vi "Nfocus driver V0.3.vi"(5 "error in":errorcluster) -> (0 "error out":errorcluster)   [LabVIEW 2016]
panel:
  in  "Refs In":T1
  out "Running":bool
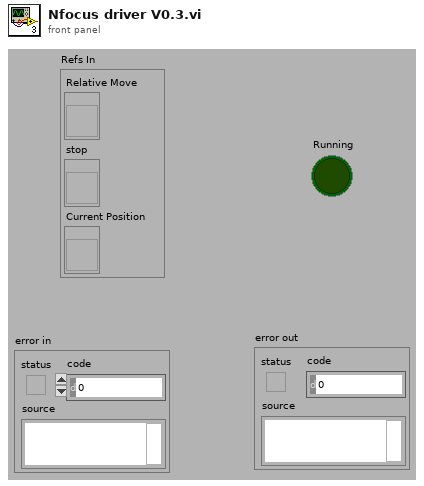
[diagram p1: front panel]
types:
  T1 = cluster{"Relative Move":refnum<vi>, "stop":refnum<vi>, "Current Position":refnum<vi>}
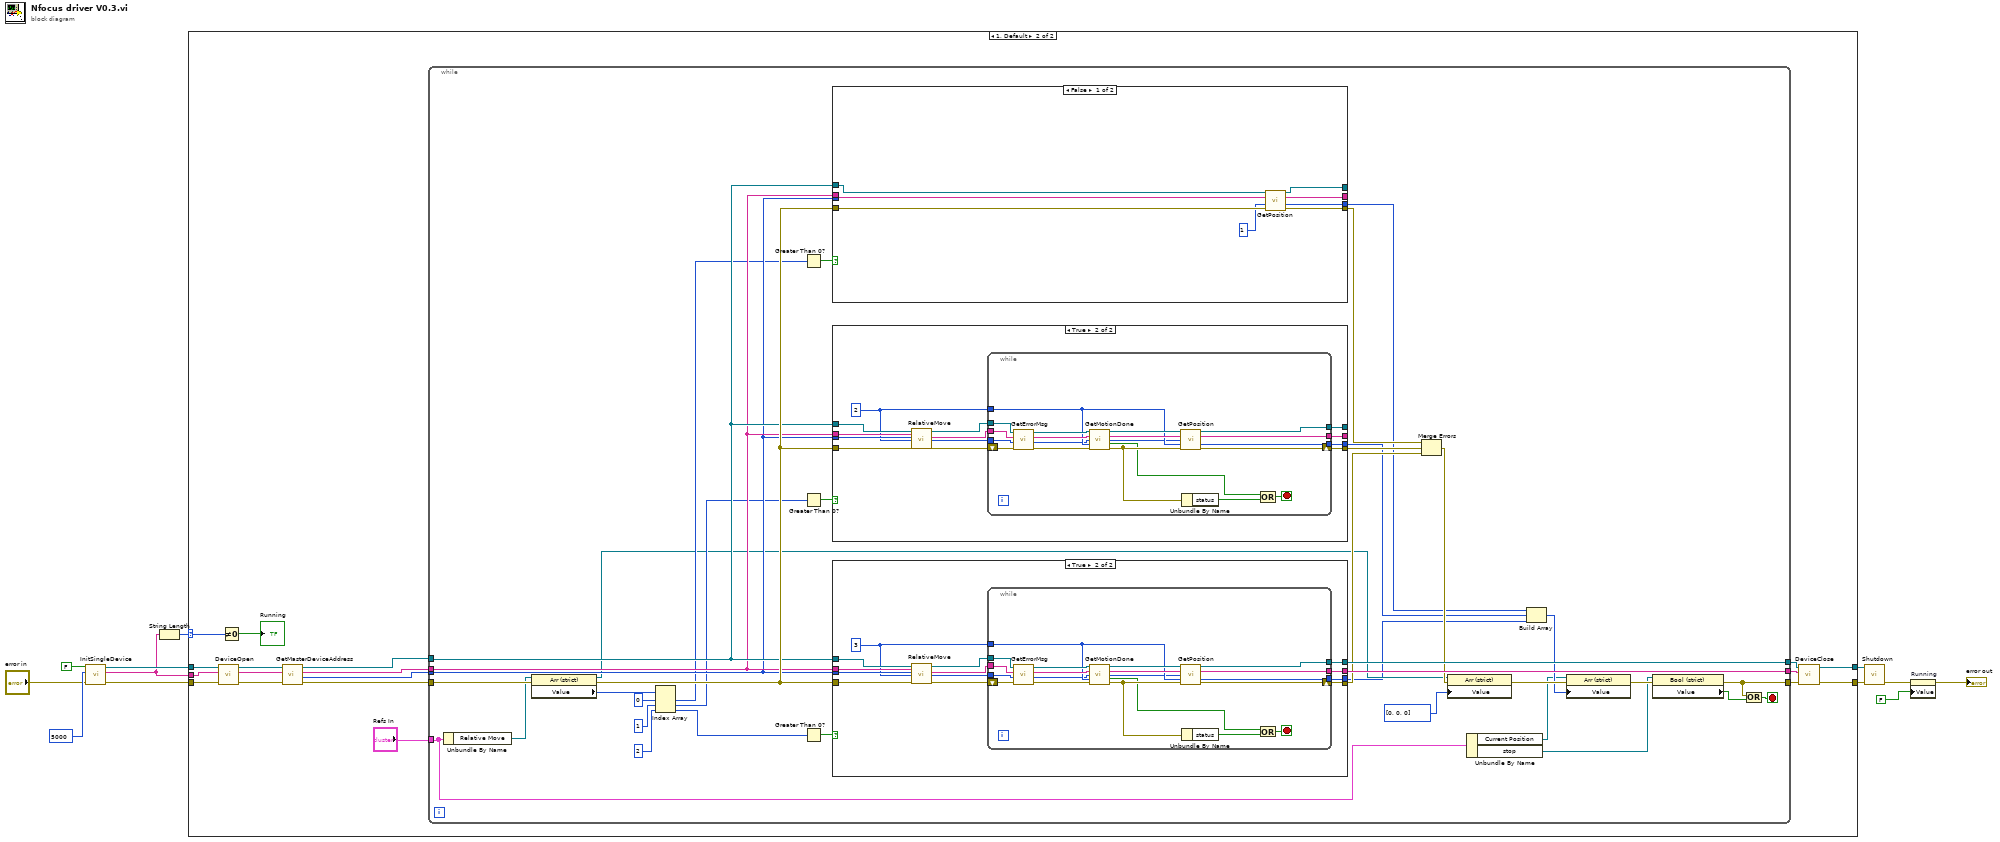
[diagram p0: block diagram]
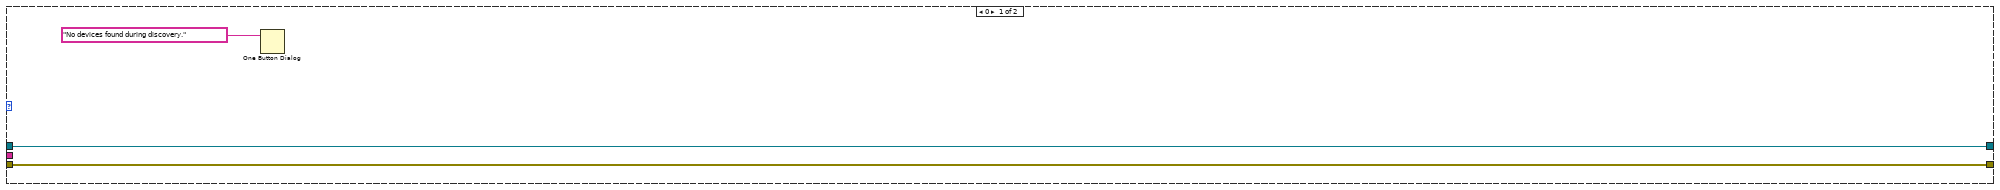
[diagram p2: hidden frame]
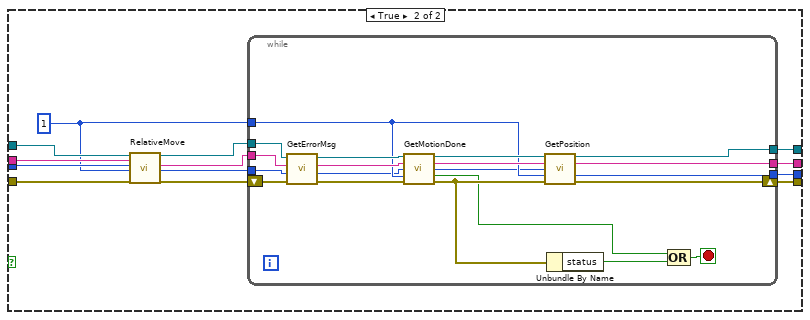
[diagram p3: hidden frame]
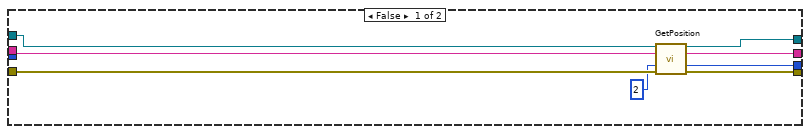
[diagram p4: hidden frame]
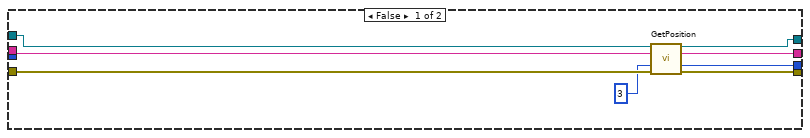
[diagram p5: hidden frame]
diagram:
  n1 = call "InitSingleDevice.vi"("error in (no error)"="error in", "msecDelayForDiscovery"=5000, "logging"=FALSE) -> ("error out"=w5:errorcluster, "DeviceKey Out"=w6:string, "CmdLib Out"=w8:refnum<k24>)  [unwired: 2 in]
  n2 = String Length(string=w6) -> (length=w7:i32)
  n3 = case shown="1, Default" w7 {
    selector: w7 -> [_ w18]
    tunnel: [w14 w20] -> w10
    tunnel: [w13 w22] -> w9
    tunnel: w8 -> [w14 w26]
    tunnel: w6 -> [_ w28]
    tunnel: w5 -> [w13 w30]
    frame 0 {
      n4 = One Button Dialog(message="No devices found during discovery.") -> ()  [unwired: 1 in, 1 out]
    }
    frame 1, Default {
      n5 = call "DeviceOpen.vi"("error in (no error)"=w30, "DeviceKey In"=w28, "CmdLib In"=w26) -> ("error out"=w29:errorcluster, "DeviceKey Out"=w27:string, "CmdLib Out"=w25:refnum<k24>)  [unwired: 2 in]
      n6 = Not Equal To 0?(x=w18) -> (x != 0?=→"Running":bool)
      n7 = call "GetMasterDeviceAddress.vi"("error in (no error)"=w29, "DeviceKey In"=w27, "CmdLib In"=w25) -> ("error out"=w19:errorcluster, "Device Address"=w33:i32, "DeviceKey Out"=w31:string, "CmdLib Out"=w32:refnum<k24>)  [unwired: 1 in]
      n8 = while {
        tunnel: w33 -> [w57]
        tunnel: w32 -> [w59]
        tunnel: [w68] -> w21
        tunnel: w19 -> [w61]
        tunnel: [w66] -> w23
        tunnel: w31 -> [w58]
        tunnel: [w69] -> w24
        tunnel: "Refs In" -> [w36]
        stop <- w67 stop-if-true
        n9 = Unbundle By Name(w36) -> ("Relative Move"=w46:refnum<vi>)
        n10 = property class="Arr (strict)"(reference=w46, error in=w61) -> (reference out=w44:refnum<vi>, error out=w60:errorcluster, "Value"=w63:i32[])
        n11 = Index Array(array=w63, index #1=0 ("index"), index #2=1 ("index"), index #3=2 ("index")) -> (element #1=w52:i32, element #2=w51:i32, element #3=w50:i32)
        n12 = Greater Than 0?(x=w52) -> (x > 0?=w53:bool)
        n13 = Greater Than 0?(x=w51) -> (x > 0?=w54:bool)
        n14 = Greater Than 0?(x=w50) -> (x > 0?=w64:bool)
        n15 = case shown="False" w53 {
          tunnel: w57 -> [_ w90]
          tunnel: w59 -> [w77 w89]
          tunnel: w58 -> [w76 w88]
          tunnel: [w73 w87] -> _
          tunnel: [w72 w86] -> _
          tunnel: w60 -> [w75 w85]
          tunnel: [w74 w84] -> w49
          tunnel: [w71 w78] -> w40
          frame False {
            n16 = call "GetPosition.vi"("CmdLib In"=w77, "DeviceKey In"=w76, "Motor"=1, "error in (no error)"=w75) -> ("CmdLib Out"=w72:refnum<k24>, "DeviceKey Out"=w73:string, "Position"=w71:i32, "error out"=w74:errorcluster)  [unwired: 7 in, 1 out]
          }
          frame True {
            w79 = 1
            n17 = call "RelativeMove.vi"("CmdLib In"=w89, "DeviceKey In"=w88, "Device Address In"=w90, "Motor"=w79, "error in (no error)"=w85) -> ("CmdLib Out"=w83:refnum<k24>, "DeviceKey Out"=w82:string, "Device Address Out"=w80:i32, "error out"=w81:errorcluster)  [unwired: 11 in]
            n18 = while {
              tunnel: w79 -> [w106]
              tunnel: w83 -> [w105]
              tunnel: w82 -> [w104]
              tunnel: [w99] -> w86
              tunnel: w80 -> [w98]
              shift-right: [w100] -> w84
              shift-left: w81 -> [w103]
              tunnel: [w95] -> w87
              tunnel: [w91] -> w78
              stop <- w94 stop-if-true
              n19 = call "GetErrorMsg.vi"("error in (no error)"=w103, "Device Address In"=w98, "DeviceKey In"=w104, "CmdLib In"=w105) -> ("error out"=w102:errorcluster, "Device Address Out"=w97:i32, "DeviceKey Out"=w108:string, "CmdLib Out"=w107:refnum<k24>)
              n20 = call "GetMotionDone.vi"("CmdLib In"=w107, "DeviceKey In"=w108, "Device Address In"=w97, "Motor"=w106, "error in (no error)"=w102) -> ("CmdLib Out"=w109:refnum<k24>, "DeviceKey Out"=w110:string, "Device Address Out"=w96:i32, "Is Motion Done"=w93:bool, "error out"=w101:errorcluster)  [unwired: 6 in]
              n21 = call "GetPosition.vi"("CmdLib In"=w109, "DeviceKey In"=w110, "Device Address In"=w96, "Motor"=w106, "error in (no error)"=w101) -> ("CmdLib Out"=w99:refnum<k24>, "DeviceKey Out"=w95:string, "Position"=w91:i32, "error out"=w100:errorcluster)  [unwired: 6 in, 1 out]
              n22 = Unbundle By Name(w101) -> ("status"=w92:bool)
              n23 = Compound Arithmetic op=OR(w93, w92) -> (w94:bool)
            }
          }
        }
        n24 = case shown="True" w54 {
          tunnel: w57 -> [_ w131]
          tunnel: w59 -> [w118 w130]
          tunnel: w58 -> [w117 w129]
          tunnel: [w114 w128] -> _
          tunnel: [w115 w127] -> _
          tunnel: w60 -> [w116 w126]
          tunnel: [w113 w125] -> w48
          tunnel: [w111 w119] -> w39
          frame False {
            n25 = call "GetPosition.vi"("CmdLib In"=w118, "DeviceKey In"=w117, "Motor"=2, "error in (no error)"=w116) -> ("CmdLib Out"=w115:refnum<k24>, "DeviceKey Out"=w114:string, "Position"=w111:i32, "error out"=w113:errorcluster)  [unwired: 7 in, 1 out]
          }
          frame True {
            w120 = 2
            n26 = call "RelativeMove.vi"("CmdLib In"=w130, "DeviceKey In"=w129, "Device Address In"=w131, "Motor"=w120, "error in (no error)"=w126) -> ("CmdLib Out"=w124:refnum<k24>, "DeviceKey Out"=w123:string, "Device Address Out"=w121:i32, "error out"=w122:errorcluster)  [unwired: 11 in]
            n27 = while {
              tunnel: w120 -> [w147]
              tunnel: w124 -> [w146]
              tunnel: w123 -> [w145]
              tunnel: [w140] -> w127
              tunnel: w121 -> [w139]
              shift-right: [w141] -> w125
              shift-left: w122 -> [w144]
              tunnel: [w136] -> w128
              tunnel: [w132] -> w119
              stop <- w135 stop-if-true
              n28 = call "GetErrorMsg.vi"("error in (no error)"=w144, "Device Address In"=w139, "DeviceKey In"=w145, "CmdLib In"=w146) -> ("error out"=w143:errorcluster, "Device Address Out"=w138:i32, "DeviceKey Out"=w149:string, "CmdLib Out"=w148:refnum<k24>)
              n29 = call "GetMotionDone.vi"("CmdLib In"=w148, "DeviceKey In"=w149, "Device Address In"=w138, "Motor"=w147, "error in (no error)"=w143) -> ("CmdLib Out"=w150:refnum<k24>, "DeviceKey Out"=w151:string, "Device Address Out"=w137:i32, "Is Motion Done"=w134:bool, "error out"=w142:errorcluster)  [unwired: 6 in]
              n30 = call "GetPosition.vi"("CmdLib In"=w150, "DeviceKey In"=w151, "Device Address In"=w137, "Motor"=w147, "error in (no error)"=w142) -> ("CmdLib Out"=w140:refnum<k24>, "DeviceKey Out"=w136:string, "Position"=w132:i32, "error out"=w141:errorcluster)  [unwired: 6 in, 1 out]
              n31 = Unbundle By Name(w142) -> ("status"=w133:bool)
              n32 = Compound Arithmetic op=OR(w134, w133) -> (w135:bool)
            }
          }
        }
        n33 = case shown="True" w64 {
          tunnel: w57 -> [_ w172]
          tunnel: w59 -> [w159 w171]
          tunnel: w58 -> [w158 w170]
          tunnel: [w155 w169] -> w69
          tunnel: [w154 w168] -> w68
          tunnel: w60 -> [w157 w167]
          tunnel: [w156 w166] -> w47
          tunnel: [w152 w160] -> w38
          frame False {
            n34 = call "GetPosition.vi"("CmdLib In"=w159, "DeviceKey In"=w158, "Motor"=3, "error in (no error)"=w157) -> ("CmdLib Out"=w154:refnum<k24>, "DeviceKey Out"=w155:string, "Position"=w152:i32, "error out"=w156:errorcluster)  [unwired: 7 in, 1 out]
          }
          frame True {
            w161 = 3
            n35 = call "RelativeMove.vi"("CmdLib In"=w171, "DeviceKey In"=w170, "Device Address In"=w172, "Motor"=w161, "error in (no error)"=w167) -> ("CmdLib Out"=w165:refnum<k24>, "DeviceKey Out"=w164:string, "Device Address Out"=w162:i32, "error out"=w163:errorcluster)  [unwired: 11 in]
            n36 = while {
              tunnel: w161 -> [w188]
              tunnel: w165 -> [w187]
              tunnel: w164 -> [w186]
              tunnel: [w181] -> w168
              tunnel: w162 -> [w180]
              shift-right: [w182] -> w166
              shift-left: w163 -> [w185]
              tunnel: [w177] -> w169
              tunnel: [w173] -> w160
              stop <- w176 stop-if-true
              n37 = call "GetErrorMsg.vi"("error in (no error)"=w185, "Device Address In"=w180, "DeviceKey In"=w186, "CmdLib In"=w187) -> ("error out"=w184:errorcluster, "Device Address Out"=w179:i32, "DeviceKey Out"=w190:string, "CmdLib Out"=w189:refnum<k24>)
              n38 = call "GetMotionDone.vi"("CmdLib In"=w189, "DeviceKey In"=w190, "Device Address In"=w179, "Motor"=w188, "error in (no error)"=w184) -> ("CmdLib Out"=w191:refnum<k24>, "DeviceKey Out"=w192:string, "Device Address Out"=w178:i32, "Is Motion Done"=w175:bool, "error out"=w183:errorcluster)  [unwired: 6 in]
              n39 = call "GetPosition.vi"("CmdLib In"=w191, "DeviceKey In"=w192, "Device Address In"=w178, "Motor"=w188, "error in (no error)"=w183) -> ("CmdLib Out"=w181:refnum<k24>, "DeviceKey Out"=w177:string, "Position"=w173:i32, "error out"=w182:errorcluster)  [unwired: 6 in, 1 out]
              n40 = Unbundle By Name(w183) -> ("status"=w174:bool)
              n41 = Compound Arithmetic op=OR(w175, w174) -> (w176:bool)
            }
          }
        }
        n42 = Merge Errors(w49, w48, w47) -> (w45:errorcluster)
        n43 = property class="Arr (strict)"(reference=w44, error in=w45, "Value"=i32[] [0, 0, 0]) -> (error out=w42:errorcluster)  [unwired: 1 out]
        n44 = Unbundle By Name(w36) -> ("Current Position"=w35:refnum<vi>, "stop"=w34:refnum<vi>)
        n45 = Build Array(w40, w39, w38) -> (w37:i32[])
        n46 = property class="Arr (strict)"(reference=w35, error in=w42, "Value"=w37) -> (error out=w41:errorcluster)  [unwired: 1 out]
        n47 = property on="Property Node" class="Bool (strict)"(reference=w34, error in=w41) -> (error out=w66:errorcluster, "Value"=w65:bool)  [unwired: 1 out]
        n48 = Compound Arithmetic op=OR(w66, w65) -> (w67:bool)
      }
      n49 = call "DeviceClose.vi"("error in (no error)"=w23, "DeviceKey In"=w24, "CmdLib In"=w21) -> ("error out"=w22:errorcluster, "CmdLib Out"=w20:refnum<k24>)  [unwired: 2 in, 1 out]
    }
  }
  n50 = call "Shutdown.vi"("error in (no error)"=w9, "CmdLib In"=w10) -> ("error out"=w3:errorcluster)  [unwired: 4 in, 1 out]
  n51 = property on="Running" class="Bool (strict)"(error in=w3, "Value"=FALSE ("Boolean")) -> (error out=→"error out":errorcluster)  [unwired: 1 in, 1 out]
